vi "array2Img (SubVI).vi"(11 "Rxy":dbl[][](array[numeric])) -> (3 "new picture":picture)   [LabVIEW 2014]
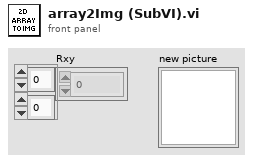
[diagram p1: front panel]
types:
  T1 = typedef "imagedata.ctl" = cluster{"image type":i32, "image depth":i32, "image":u8[], "mask":u8[], "colors":u32[], "Rectangle":cluster{"left":i16, "top":i16, "right":i16, "bottom":i16}}
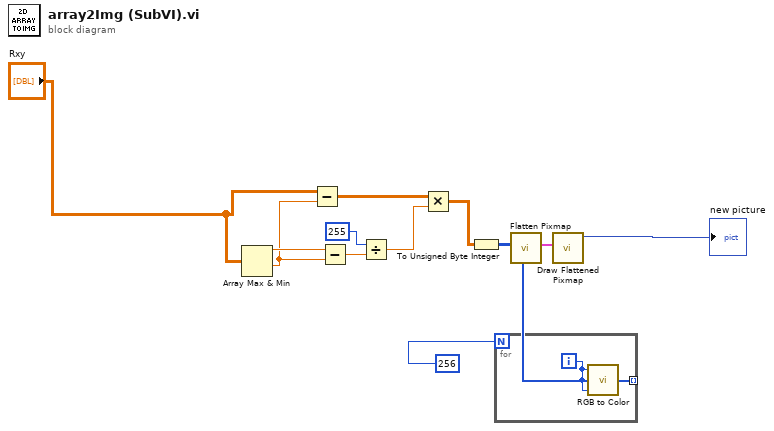
[diagram p0: block diagram]
diagram:
  n1 = Array Max & Min(array="Rxy") -> (max value=w3:dbl, min value=w2:dbl)  [unwired: 2 out]
  n2 = Subtract(x="Rxy", y=w2) -> (x-y=w5:dbl[][])
  n3 = Subtract(x=w3, y=w2) -> (x-y=w6:dbl)
  n4 = Divide(x=u8 255, y=w6) -> (x/y=w7:dbl)
  n5 = Multiply(x=w5, y=w7) -> (x*y=w1:dbl[][])
  n6 = To Unsigned Byte Integer(number=w1) -> (unsigned 8bit integer=w11:u8[][])
  n7 = for {
    N: 256 -> [_]
    tunnel: [w14] -> w13 mode=indexing
    i -> [w15]
    n8 = call <vilib>:"RGB to Color.vi"("B"=w15, "G"=w15, "R"=w15) -> ("Color"=w14:u32)
  }
  n9 = call <vilib>:"Flatten Pixmap.vi"("colors"=w13, "8-bit pixmap"=w11) -> ("image data"=w10:T1)  [unwired: 9 in]
  n10 = call <vilib>:"Draw Flattened Pixmap.vi"("image data"=w10) -> ("new picture"=→"new picture":picture)  [unwired: 8 in]
